vi "Suggested Troubleshooting from R&D.vi"() -> ()   [LabVIEW 2014]
uses:
  Controls/States.ctl
panel:
  in  "Suggested Troubleshooting from R&D":T2(array[cluster])
  # "Suggested Troubleshooting from R&D"
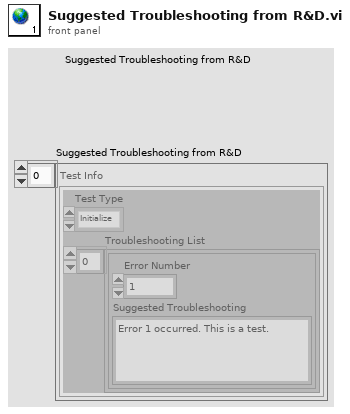
[diagram p1: front panel]
types:
  T1 = typedef "States.ctl" = enum16{"Initialize", "Wait for User Input", "Check User Input", "Insert Open VI", "Run Open VI", "Straight Line", "Home", "Limit", "Generate Report", "Finalize", "Terminate"}
  T2 = cluster{"Test Type":T1, "Troubleshooting List":cluster{"Error Number":i32, "Suggested Troubleshooting":string}[]}[]
diagram:
